vi "Data_Brekadown_OE_cal.vi"(7 "Refnum in":T1, 8 "error in (no error)":errorcluster, 9 "Station No":i32, 10 "Date":timestamp, 11 "Shift":string) -> (0 "error out":errorcluster, 3 "Break_down_Data":string[][](array[string]))   [LabVIEW 2017]
uses:
  <vilib>/addons/database/Connection.llb/Conn ObjectReference.ctl
  <vilib>/addons/database/_DB Variant To Data/Database Variant To Data.xnode
  <vilib>/addons/database/NI_Database_API.lvlib
panel:
  out "resulting string":string
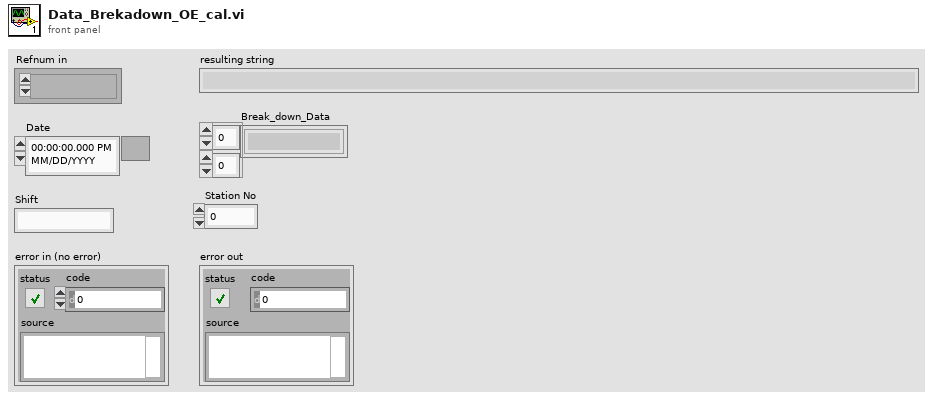
[diagram p1: front panel]
types:
  T1 = typedef "NI_Database_API.lvlib/Conn ObjectReference.ctl" = refnum<k1>
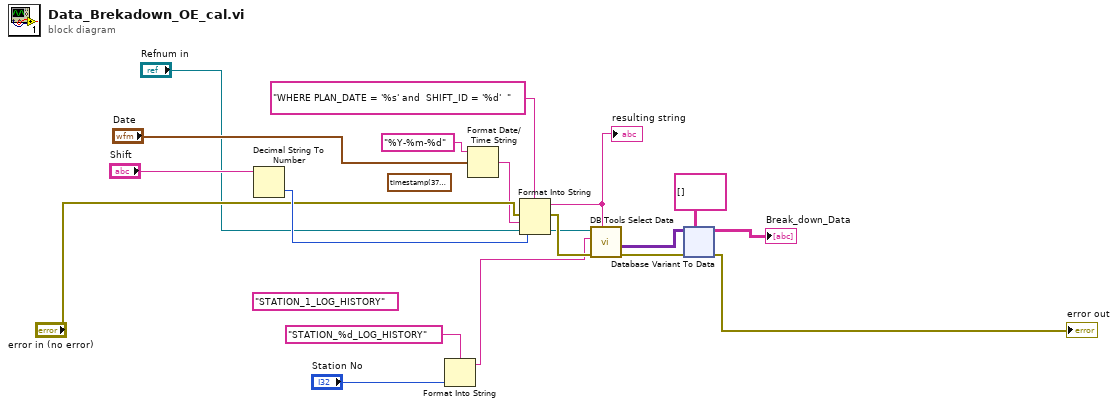
[diagram p0: block diagram]
diagram:
  (unwired) timestamp(3772310400 s since 1904-01-01) ("Date")
  (unwired) "STATION_1_LOG_HISTORY" ("table")
  n1 = Decimal String To Number(string="Shift") -> (number=w17:i32)  [unwired: 2 in, 1 out]
  n2 = Format Into String(format string="STATION_%d_LOG_HISTORY" ("table"), "Station No") -> (resulting string=w1:string)  [unwired: 2 in, 1 out]
  n3 = Format Date/Time String(time format string (%c)="%Y-%m-%d", seconds (now)="Date") -> (date/time string=w11:string)  [unwired: 1 in]
  n4 = Format Into String(format string="WHERE PLAN_DATE = '%s' and  SHIFT_ID = '%d'  ", error in="error in (no error)", w11, w17) -> (resulting string=w13:string, error out=w16:errorcluster)  [unwired: 1 in]
  "resulting string" <- w13
  n5 = call <vilib>:"DB Tools Select Data.vi"("condition"=w13, "error in (no error)"=w16, "table"=w1, "connection reference"="Refnum in") -> ("error out"=w5:errorcluster, "data"=w6:variant[][])  [unwired: 2 in, 1 out]
  n6 = xnode "Database Variant To Data"("database variant"=w6, "error in (no error)"=w5, "type"=string[][] [] ("Elements Found")) -> ("data"=→"Break_down_Data":string[][], "error out"=→"error out":errorcluster)
